vi "DealDataFinalVersion.vi"(0 "ArrayIn":u8[](array[numeric])=[0, 0, 0, 0, 0, 0, 0, 0, 0, 0, 0, 0, 0, 0, 0, 0, 0, 0, 0, 0, 0, 0, 0, 0, 0, 0, 0, 0, 0, 0, 0, 0, 0, 0, 0, 0, 0, 0, 0, 0, 0, 0, 0, 0, 0, 0, 0, 0, 0, 0, 0, 0, 0, 0, 0, 0, 0, 0, 0, 0, 0, 0, 0, 0, 0, 0, 0, 0, 0, 0, 0, 0, 0, 0, 0, 0, 0, 0, 0, 0, 0, 0, 0, 0, 0, 0, 0, 0, 0, 0, 0, 0, 0, 0, 0, 0, 0, 0, 0, 0, 0, 0, 0, 0, 0, 0, 0, 0, 0, 0, 0, 0, 0, 0, 0, 0, 0, 0, 0, 0, 0, 0, 0, 0, 0, 0, 0, 0, 0, 0, 0, 0, 0, 0, 0, 0, 0, 0, 0, 0, 0, 0] format="0x%x", 2 "确定按钮":bool) -> (1 "输出数组":string[][](array[string]))   [LabVIEW 2011]
panel:
  out "数组 4":i32[](array[numeric])
  out "数组 3":u8[](array[numeric])
  out "数组 2":u8[](array[numeric])
  out "数组":u8[](array[numeric])
  out "stringTwo":string[](array[string])
  out "stringOne":string[](array[string])
  out "mu08CountNumArrayIndex":u8
  out "mu08BufSize":u8
  # "将获取的数据，根据协议内部的数据长度进行数据分析"
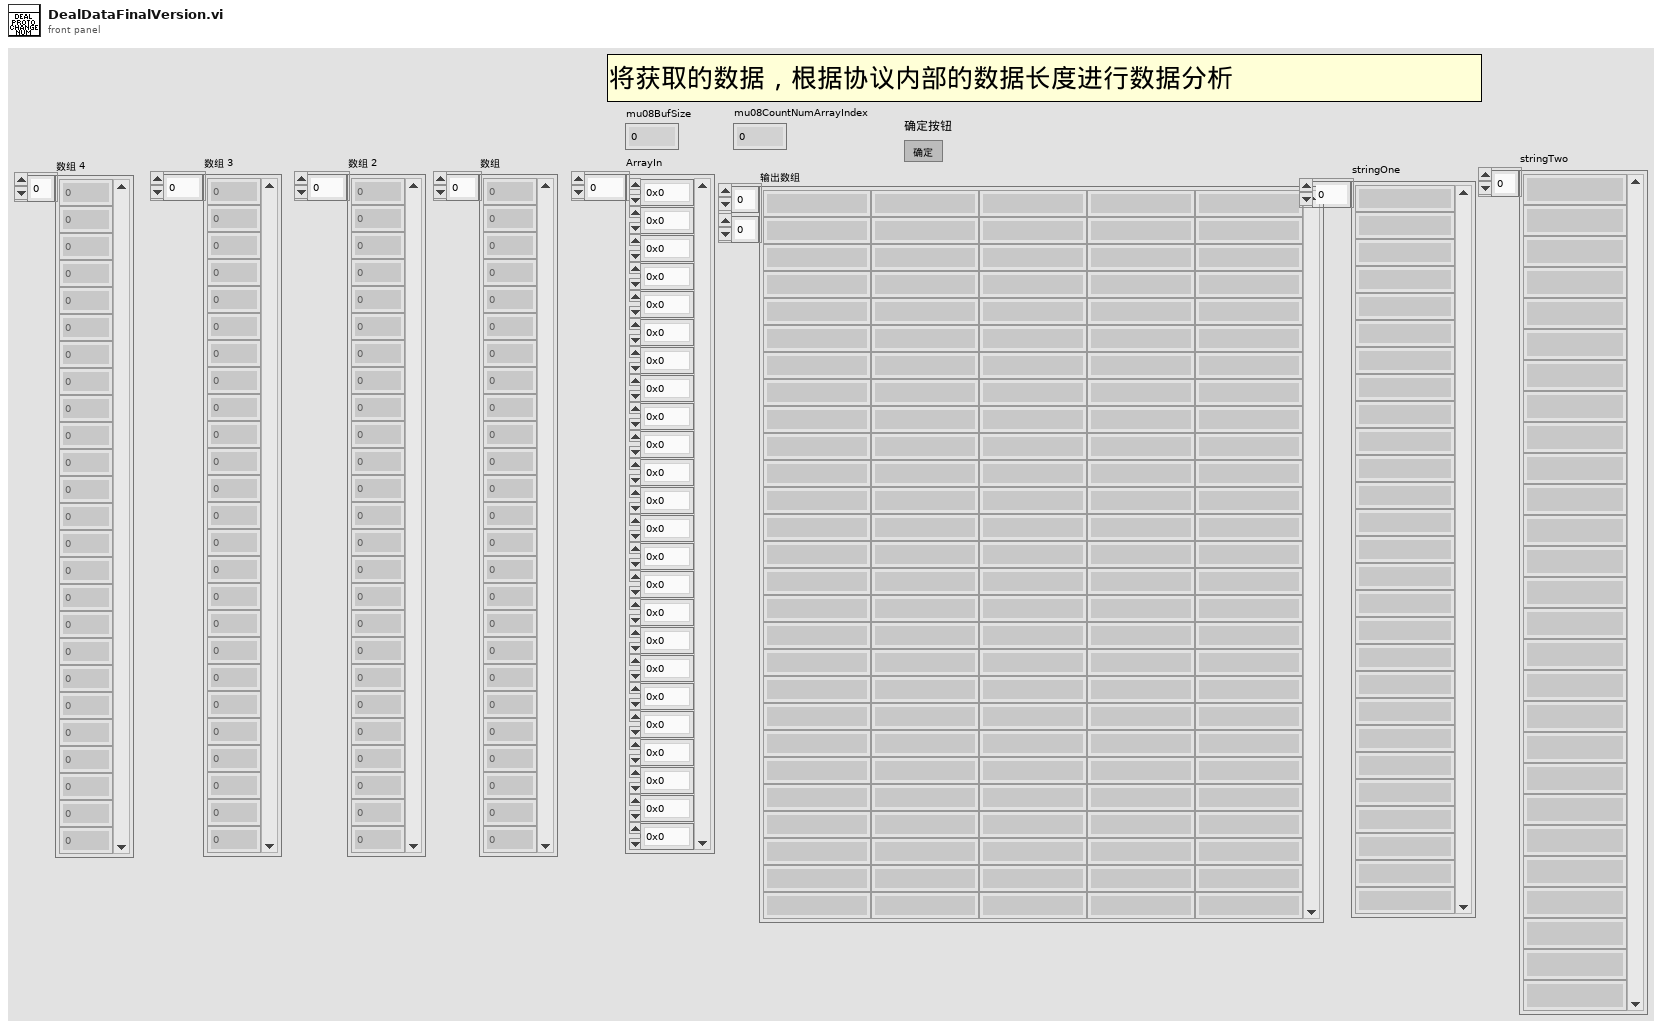
[diagram p1: front panel]
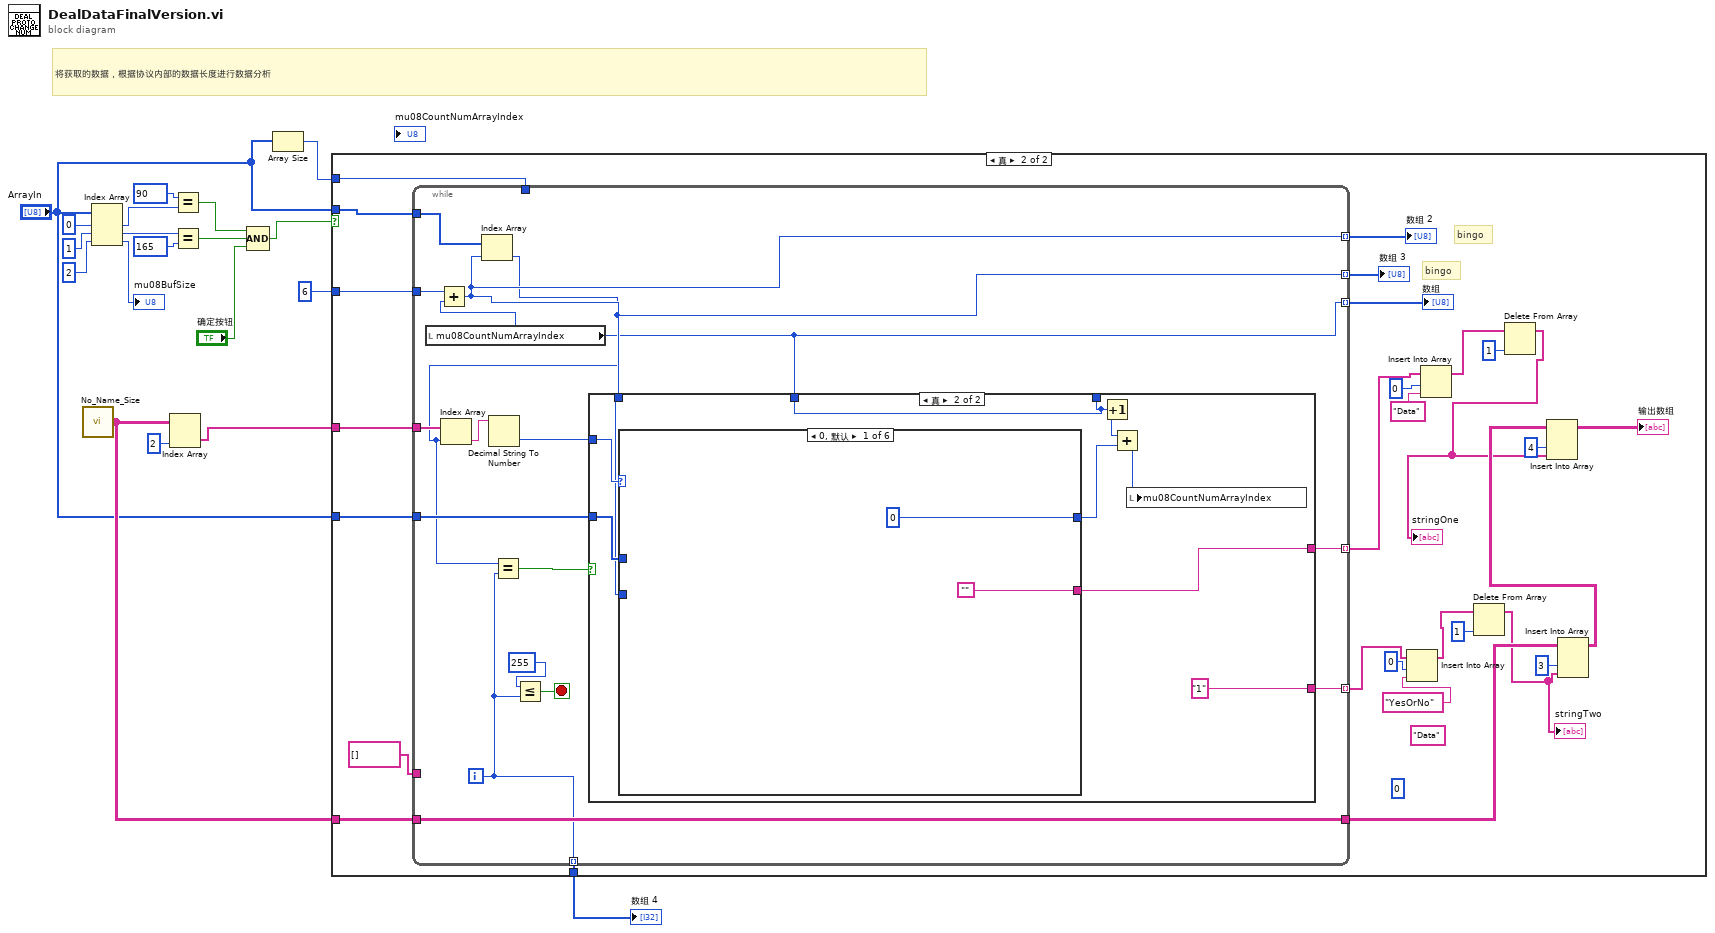
[diagram p0: block diagram]
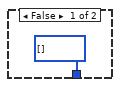
[diagram p2: hidden frame]
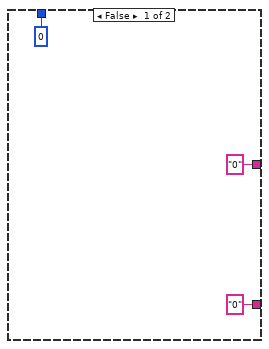
[diagram p3: hidden frame]
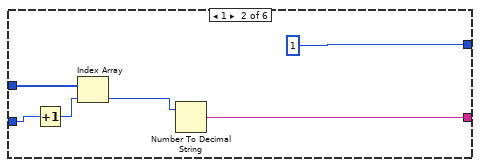
[diagram p4: hidden frame]
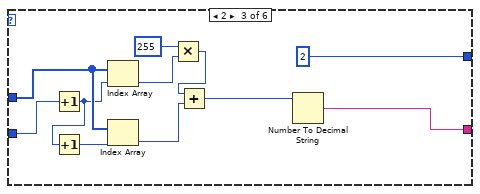
[diagram p5: hidden frame]
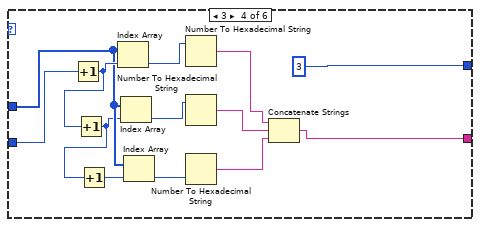
[diagram p6: hidden frame]
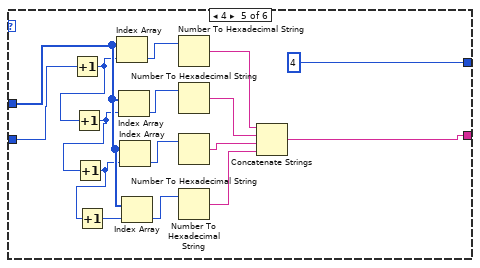
[diagram p7: hidden frame]
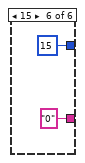
[diagram p8: hidden frame]
diagram:
  # "将获取的数据，根据协议内部的数据长度进行数据分析"
  n1 = call "No_Name_Size.vi"() -> ("数组"=w6:string[][])
  n2 = Index Array(array="ArrayIn", index #1=0 ("索引"), index #2=1 ("索引"), index #3=2 ("索引")) -> (element #1=w16:u8, element #2=w15:u8, element #3=→"mu08BufSize":u8)
  n3 = Index Array(array=w6, index (col)=2 ("禁用的索引 (列)")) -> (element=w7:string[])  [unwired: 1 in]
  n4 = Equal?(x=u8 90, y=w16) -> (x = y?=w12:bool)
  n5 = Equal?(x=w15, y=u8 165 ("x")) -> (x = y?=w11:bool)
  n6 = Compound Arithmetic op=AND(w12, w11, "确定按钮") -> (w10:bool)
  n7 = Array Size(array="ArrayIn") -> (size(s)=w3:i32)
  n8 = case shown="真" w10 {
    tunnel: 6 -> [_ w47]
    tunnel: "ArrayIn" -> [_ w48]
    tunnel: w7 -> [_ w46]
    tunnel: "ArrayIn" -> [_ w45]
    tunnel: w6 -> [_ w44]
    tunnel: [i32[] [] w30] -> w5
    tunnel: w3 -> [_ w27]
    frame False {
    }
    frame True {
      (unwired) "Data"
      (unwired) 0 ("索引")
      # "bingo"
      # "bingo"
      n9 = while {
        tunnel: w48 -> [w64]
        tunnel: w47 -> [w63]
        tunnel: w46 -> [w62]
        tunnel: w45 -> [w57]
        tunnel: [w58] -> w39
        tunnel: w44 -> [w58]
        tunnel: [w54] -> w37 mode=indexing
        tunnel: [w56] -> w35 mode=indexing
        tunnel: [w52] -> w34 mode=indexing
        tunnel: [w55] -> w33 mode=indexing
        tunnel: [w51] -> w32 mode=indexing
        tunnel: string[] [] ("数组") -> [_]
        tunnel: [w50] -> w30 mode=indexing
        tunnel: w27 -> [_]
        i -> [w50]
        stop <- w59 stop-if-true
        n10 = local read "mu08CountNumArrayIndex"() -> (w52:u8)
        n11 = Add(x=w63, y=w52) -> (x+y=w55:i32)
        n12 = Index Array(array=w64, index=w55) -> (element=w51:u8)
        n13 = Index Array(array=w62, index=w51) -> (element=w61:string)
        n14 = Decimal String To Number(string=w61) -> (number=w60:i32)  [unwired: 2 in, 1 out]
        n15 = Equal?(x=w51, y=w50) -> (x = y?=w53:bool)
        n16 = Less Or Equal?(x=255, y=w50) -> (x <= y?=w59:bool)
        n17 = case shown="真" w53 {
          tunnel: w60 -> [_ w76]
          tunnel: w57 -> [_ w73]
          tunnel: ["0" ("新元素/子数组") "1" ("新元素/子数组")] -> w56
          tunnel: w55 -> [_ w71]
          tunnel: ["0" w70] -> w54
          tunnel: [u8 0 ("mu08CountNumArrayIndex") w68] -> _
          tunnel: w52 -> [_ w68]
          frame False {
          }
          frame True {
            n18 = case shown="0, 默认" w76 {
              tunnel: [0 1 2 3 4 15] -> w69
              tunnel: w73 -> [_ w83 w94 w106 w123 _]
              tunnel: w71 -> [_ w81 w91 w103 w118 _]
              tunnel: ["" w79 w85 w96 w109 "0"] -> w70
              frame 0, Default {
              }
              frame 1 {
                n19 = Increment(x=w81) -> (x+1=w82:i32)
                n20 = Index Array(array=w83, index=w82) -> (element=w80:u8)
                n21 = Number To Decimal String(number=w80) -> (decimal integer string=w79:string)  [unwired: 1 in]
              }
              frame 2 {
                n22 = Increment(x=w91) -> (x+1=w93:i32)
                n23 = Increment(x=w93) -> (x+1=w92:i32)
                n24 = Index Array(array=w94, index=w93) -> (element=w90:u8)
                n25 = Index Array(array=w94, index=w92) -> (element=w87:u8)
                n26 = Multiply(x=u16 255, y=w90) -> (x*y=w88:u16)
                n27 = Add(x=w88, y=w87) -> (x+y=w86:u16)
                n28 = Number To Decimal String(number=w86) -> (decimal integer string=w85:string)  [unwired: 1 in]
              }
              frame 3 {
                n29 = Increment(x=w103) -> (x+1=w107:i32)
                n30 = Increment(x=w107) -> (x+1=w105:i32)
                n31 = Increment(x=w105) -> (x+1=w104:i32)
                n32 = Index Array(array=w106, index=w107) -> (element=w102:u8)
                n33 = Index Array(array=w106, index=w105) -> (element=w101:u8)
                n34 = Index Array(array=w106, index=w104) -> (element=w100:u8)
                n35 = Number To Hexadecimal String(2:w102) -> (0:w99:string)  [unwired: 1 in]
                n36 = Number To Hexadecimal String(2:w101) -> (0:w98:string)  [unwired: 1 in]
                n37 = Number To Hexadecimal String(2:w100) -> (0:w97:string)  [unwired: 1 in]
                n38 = Concatenate Strings(w99, w98, w97) -> (w96:string)
              }
              frame 4 {
                n39 = Increment(x=w118) -> (x+1=w122:i32)
                n40 = Increment(x=w122) -> (x+1=w121:i32)
                n41 = Increment(x=w121) -> (x+1=w120:i32)
                n42 = Increment(x=w120) -> (x+1=w119:i32)
                n43 = Index Array(array=w123, index=w122) -> (element=w117:u8)
                n44 = Index Array(array=w123, index=w121) -> (element=w116:u8)
                n45 = Index Array(array=w123, index=w120) -> (element=w115:u8)
                n46 = Index Array(array=w123, index=w119) -> (element=w114:u8)
                n47 = Number To Hexadecimal String(2:w117) -> (0:w113:string)  [unwired: 1 in]
                n48 = Number To Hexadecimal String(2:w116) -> (0:w112:string)  [unwired: 1 in]
                n49 = Number To Hexadecimal String(2:w115) -> (0:w111:string)  [unwired: 1 in]
                n50 = Number To Hexadecimal String(2:w114) -> (0:w110:string)  [unwired: 1 in]
                n51 = Concatenate Strings(w113, w112, w111, w110) -> (w109:string)
              }
              frame 15 {
              }
            }
            n52 = Increment(x=w68) -> (x+1=w74:u8)
            n53 = Add(x=w74, y=w69) -> (x+y=w75:i32)
            n54 = local write "mu08CountNumArrayIndex"(w75) -> ()
          }
        }
      }
      "数组" <- w34
      "数组 2" <- w33
      "数组 3" <- w32
      n55 = Insert Into Array(array=w35, index=0 ("索引"), new element="YesOrNo") -> (w22:string[])
      n56 = Insert Into Array(array=w37, index=0 ("索引"), new element="Data") -> (w25:string[])
      n57 = Delete From Array(array=w22, index=1 ("索引")) -> (array with subset deleted=w21:string[])  [unwired: 1 in, 1 out]
      "stringTwo" <- w21
      n58 = Delete From Array(array=w25, index=1 ("索引")) -> (array with subset deleted=w24:string[])  [unwired: 1 in, 1 out]
      "stringOne" <- w24
      n59 = Insert Into Array(array=w39, index (col)=3 ("索引 (列)"), new element=w21) -> (w43:string[][])  [unwired: 1 in]
      n60 = Insert Into Array(array=w43, index (col)=4 ("禁用的索引 (列)"), new element=w24) -> (→"输出数组":string[][])  [unwired: 1 in]
    }
  }
  "数组 4" <- w5
